vi "pmu_Build Data Width (Std 2011).vi"(8 "error in (no error)":errorcluster, 11 "system info in":refnum<class "PMU System Info.lvclass">) -> (0 "error out":errorcluster, 2 "init meas data":u8[](array[numeric]), 3 "system info out":refnum<class "PMU System Info.lvclass">)   [LabVIEW 2013, in "NI_EP_PMU.lvlib"]
uses:
  <vilib>/addons/Electrical Power/PMU/NI_EP_PMU.lvlib
  <vilib>/addons/Electrical Power/PMU/Common/Classes/PMU System Info/PMU System Info.lvclass
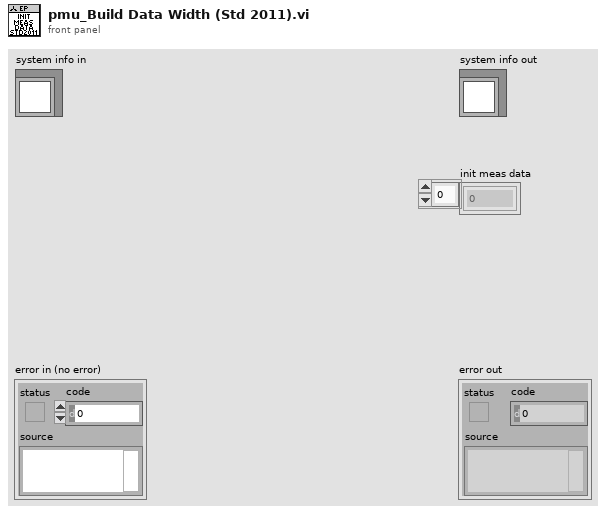
[diagram p1: front panel]
types:
  T1 = typedef "NI_EP_PMU.lvlib/pmu_CFG for Data Frame.ctl" = enum8{"CFG-2", "CFG-3"}
  T2 = typedef "NI_EP_PMU.lvlib/pmu_CFG Class.ctl" = cluster{"station name":string, "PMU ID":u16, "time base":u32, "nominal frequency":enum16{"50 Hz", "60 Hz"}, "reporting rate":i16, "phasor number":u16, "analog number":u16, "digital number":u16, "channel names":string[], "phasor units":u32[], "analog units":u32[], "digital units":u32[], "data format":u16, "number of PMUs":u16}
  T3 = typedef "pmu_CFG-3 Class.ctl" = cluster{"station name":string, "PMU ID":u16, "global PMU ID":u64, "time base":u32, "nominal frequency":enum16{"50 Hz", "60 Hz"}, "reporting rate":i16, "phasor number":u16, "analog number":u16, "digital number":u16, "channel names":string[], "phasor scale first 4 bytes":u32[], "phasor scale factors":sgl[], "phasor angle offsets [rad]":sgl[], "analog scale factors":sgl[], "analog magnitude offsets":sgl[], "digital units":u32[], "data format":u16, "number of PMUs":u16}
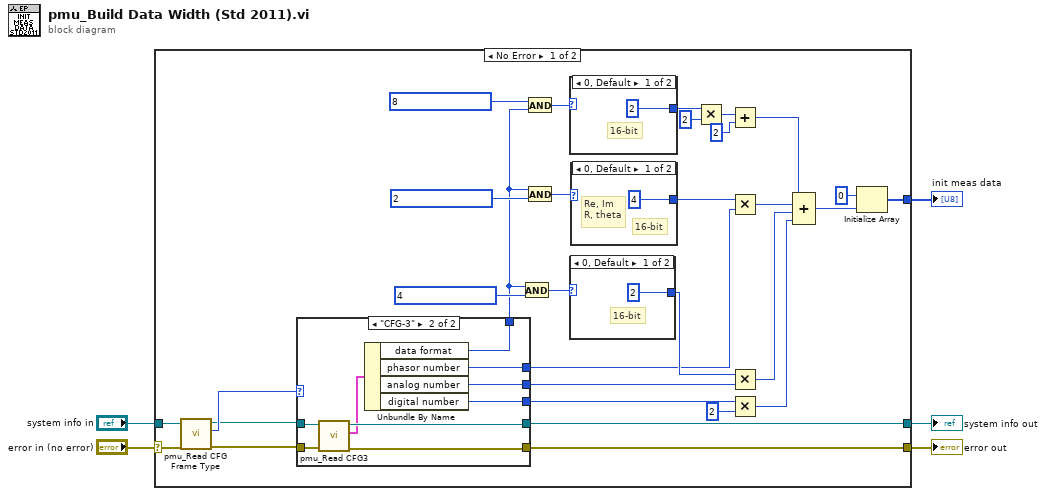
[diagram p0: block diagram]
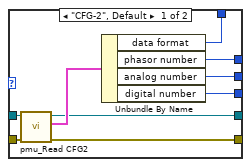
[diagram p2: hidden frame]
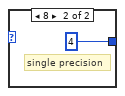
[diagram p3: hidden frame]
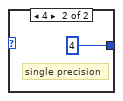
[diagram p4: hidden frame]
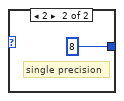
[diagram p5: hidden frame]
diagram:
  n1 = case shown="No Error" "error in (no error)" {
    selector: "error in (no error)" -> [w10 w61]
    tunnel: "system info in" -> [w6 w62]
    tunnel: [w15 w61] -> w4
    tunnel: [w14 w62] -> w3
    tunnel: [w11 _] -> w1
    frame No Error {
      n2 = call <vilib>:"pmu_Read CFG Frame Type.vi"("error in (no error)"=w10, "system info in"=w6) -> ("error out"=w9:errorcluster, "configuration frame option"=w8:T1, "system info out"=w7:refnum<class "PMU System Info.lvclass">)  [unwired: 7 in]
      n3 = case shown="\"CFG-3\"" w8 {
        tunnel: w7 -> [w45 w53]
        tunnel: [w43 w49] -> w26
        tunnel: [w42 w47] -> w25
        tunnel: [w41 w48] -> w22
        tunnel: [w40 w46] -> w21
        tunnel: [w39 w51] -> w15
        tunnel: [w38 w52] -> w14
        tunnel: w9 -> [w37 w54]
        frame "CFG-2", Default {
          n4 = call <vilib>:"pmu_Read CFG2.vi"("error in (no error)"=w37, "system info in"=w45) -> ("error out"=w39:errorcluster, "CFG-2"=w44:T2, "system info out"=w38:refnum<class "PMU System Info.lvclass">)  [unwired: 7 in]
          n5 = Unbundle By Name(w44) -> ("data format"=w43:u16, "phasor number"=w41:u16, "analog number"=w42:u16, "digital number"=w40:u16)
        }
        frame "CFG-3" {
          n6 = call <vilib>:"pmu_Read CFG3.vi"("error in (no error)"=w54, "system info in"=w53) -> ("error out"=w51:errorcluster, "CFG-3"=w50:T3, "system info out"=w52:refnum<class "PMU System Info.lvclass">)  [unwired: 7 in]
          n7 = Unbundle By Name(w50) -> ("data format"=w49:u16, "phasor number"=w48:u16, "analog number"=w47:u16, "digital number"=w46:u16)
        }
      }
      n8 = And(x=w26, y=u16 4 ("x")) -> (x .and. y?=w33:u16)
      n9 = And(x=u16 8, y=w26) -> (x .and. y?=w31:u16)
      n10 = And(x=w26, y=u16 2 ("x")) -> (x .and. y?=w35:u16)
      n11 = case shown="0, Default" w31 {
        tunnel: [u16 2 u16 4] -> w30
        frame 0, Default {
          # "16-bit"
        }
        frame 8 {
          # "single precision"
        }
      }
      n12 = case shown="0, Default" w33 {
        tunnel: [u16 2 u16 4] -> w24
        frame 0, Default {
          # "16-bit"
        }
        frame 4 {
          # "single precision"
        }
      }
      n13 = case shown="0, Default" w35 {
        tunnel: [u16 4 u16 8] -> w23
        frame 0, Default {
          # "Re, Im \nR, theta"
          # "16-bit"
        }
        frame 2 {
          # "single precision"
        }
      }
      n14 = Multiply(x=w30, y=u16 2) -> (x*y=w28:u16)
      n15 = Add(x=w28, y=u16 2) -> (x+y=w19:u16)
      n16 = Multiply(x=w23, y=w22) -> (x*y=w18:u16)
      n17 = Multiply(x=w24, y=w25) -> (x*y=w16:u16)
      n18 = Multiply(x=w21, y=u16 2) -> (x*y=w17:u16)
      n19 = Compound Arithmetic op=ADD(w19, w18, w16, w17) -> (w13:u16)
      n20 = Initialize Array(u8 0 ("element"), w13) -> (w11:u8[])
    }
    frame Error {
    }
  }
  "error out" <- w4
  "system info out" <- w3
  "init meas data" <- w1
